vi "Where do VI's come from.vi"() -> ()   [LabVIEW 2015]
doc: "<<<<LabVIEW freeware>>>>\n\nFind the origin of all VIs in memory.\n\n<<<<LabVIEW freeware>>>>\n---------------------------------------\n(c) CIT Engineering NV\nKleinhoefstraat 6\nB-2440 Geel\nmailto: info@citeng.com\n---------------------------------------\nv1.1\nLV6i, 3D controls\nV1.0\nFirst release"
panel:
  in  "GetRunning":bool
  in  "Running VIs":i32(listbox)
  in  "Open":bool
  out "Current path":string
  in  "Delete":bool
  in  "Files not used in directory":i32[](listbox)
  in  "VIs":i32(listbox)
  in  "stop":bool
  in  "Paths":i32(listbox)
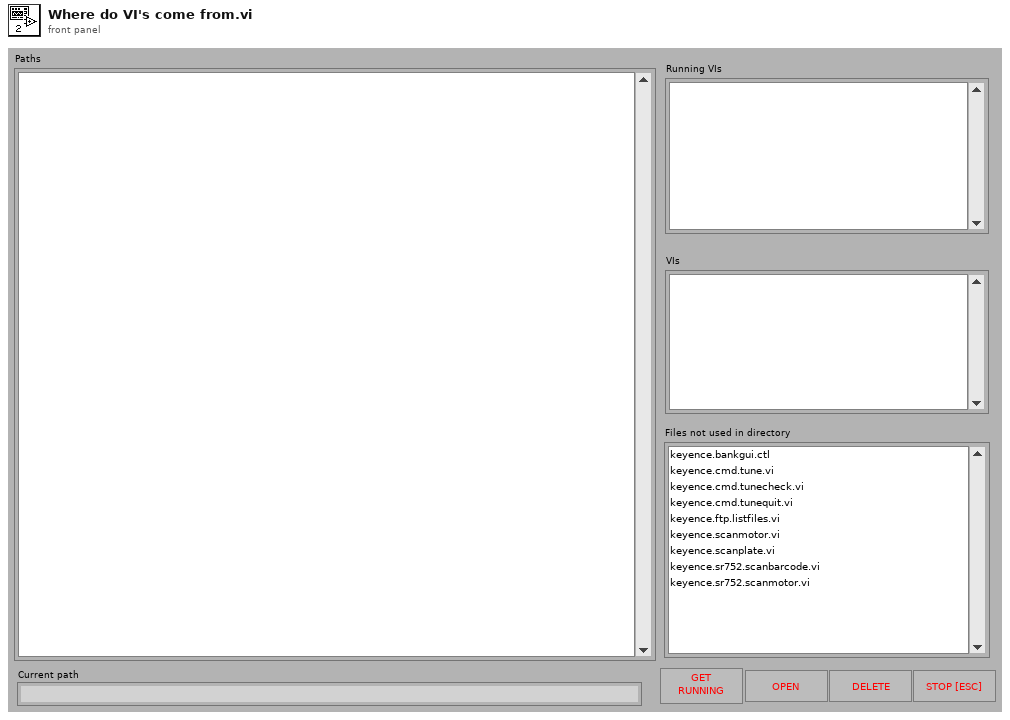
[diagram p1: front panel]
types:
  T1 = enum32{"Invalid", "Standard", "Closed", "Hidden", "Minimized", "Maximized"}
  T2 = cluster{"vi name":string, "vi path":path, "ds size":i32, "fpHeap size":i32, "bdHeap size":i32, "code size":i32, "callers":u32[], "callees":u32[]}[]
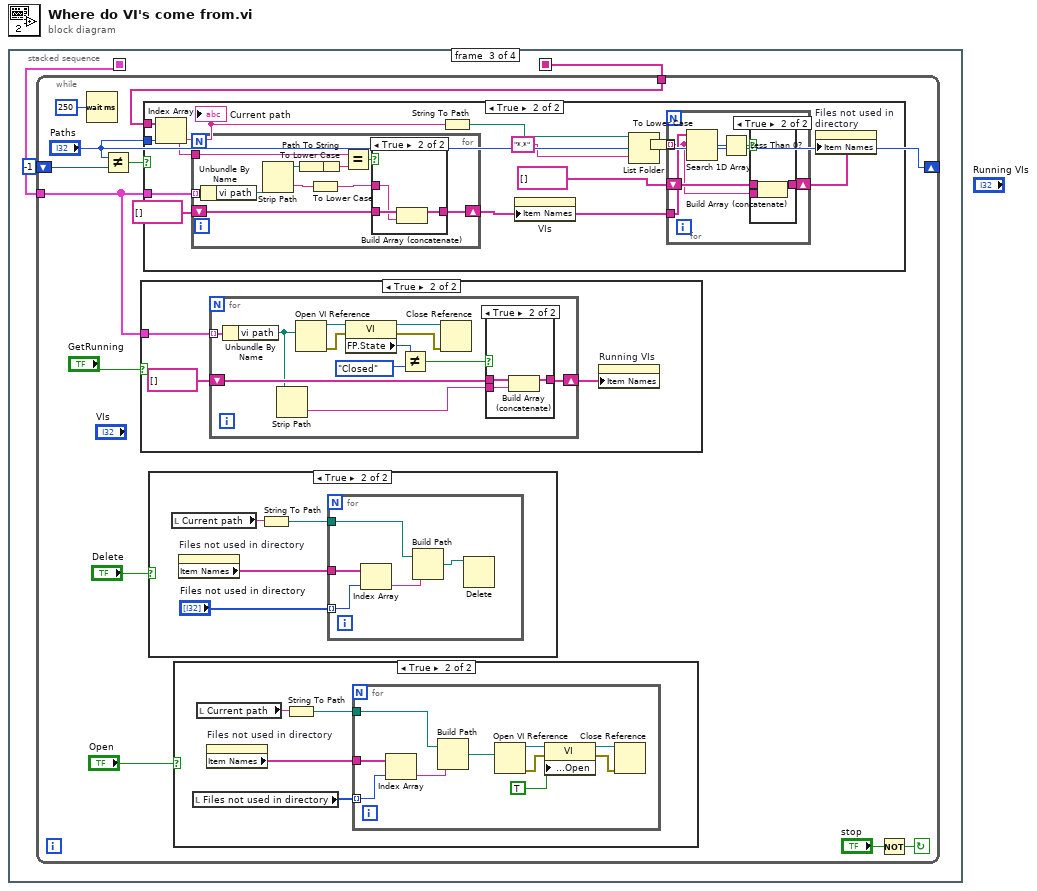
[diagram p0: block diagram]
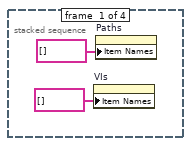
[diagram p2: hidden frame]
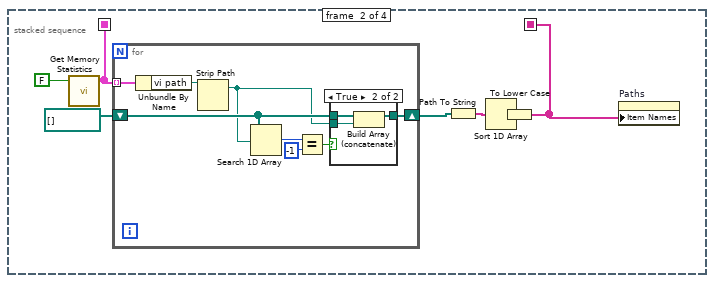
[diagram p3: hidden frame]
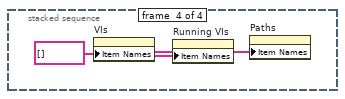
[diagram p12: hidden frame]
diagram:
  n1 = stacked-sequence {
    seq-local: [_ w3 _ _] -> [_ _ w24 _]
    seq-local: [_ w5 _ _] -> [_ _ w23 _]
    frame #0 {
      n2 = property on="VIs" class="LstBox (strict)"("Item Names"=string[] []) -> ()  [unwired: 2 in, 2 out]
      n3 = property on="Paths" class="LstBox (strict)"("Item Names"=string[] []) -> ()  [unwired: 2 in, 2 out]
    }
    frame #1 {
      n4 = call <vilib>:"Get Memory Statistics.vi"("get storage info? (T)"=FALSE) -> ("VI Memory Statistics"=w5:T2)  [unwired: 2 in, 2 out]
      n5 = for {
        tunnel: w5 -> [w17] mode=indexing
        shift-right: [w10] -> w8
        shift-left: path[] [] -> [w15]
        n6 = Unbundle By Name(w17) -> ("vi path"=w16:path)
        n7 = Strip Path(path=w16) -> (stripped path=w11:path)  [unwired: 1 out]
        n8 = Search 1D Array(1D array=w15, element=w11) -> (index of element=w14:i32)  [unwired: 1 in]
        n9 = Equal?(x=w14, y=-1) -> (x = y?=w12:bool)
        n10 = case shown="True" w12 {
          tunnel: w15 -> [w18 w21]
          tunnel: w11 -> [_ w20]
          tunnel: [w18 w19] -> w10
          frame False {
          }
          frame True {
            n11 = Build Array (concatenate)(w21, w20) -> (w19:path[])
          }
        }
      }
      n12 = Path To String(path=w8) -> (string=w7:string[])
      n13 = Sort 1D Array(array=w7) -> (sorted array=w6:string[])
      n14 = To Lower Case(string=w6) -> (all lower case string=w3:string[])
      n15 = property on="Paths" class="LstBox (strict)"("Item Names"=w3) -> ()  [unwired: 2 in, 2 out]
    }
    frame #2 {
      n16 = while {
        shift-left: -1 -> [w30]
        shift-right: ["Paths"] -> _
        tunnel: w23 -> [w26]
        tunnel: w24 -> [w33]
        stop <- w34 continue-if-true
        n17 = Wait (ms)(milliseconds to wait=u32 250) -> ()  [unwired: 1 out]
        n18 = Not Equal?(x="Paths", y=w30) -> (x != y?=w29:bool)
        n19 = case shown="True" "GetRunning" {
          tunnel: w26 -> [_ w36]
          frame False {
          }
          frame True {
            n20 = for {
              tunnel: w36 -> [w46] mode=indexing
              shift-right: [w39] -> w38
              shift-left: string[] [] -> [w45]
              n21 = Unbundle By Name(w46) -> ("vi path"=w41:path)
              n22 = Strip Path(path=w41) -> (name=w40:string)  [unwired: 1 out]
              n23 = Open VI Reference(vi path=w41) -> (vi reference=w50:refnum<vi>, error out=w49:errorcluster)  [unwired: 5 in]
              n24 = property class="VI"(reference=w50, error in=w49) -> (reference out=w47:refnum<vi>, error out=w48:errorcluster, "FP.State"=w44:T1)
              n25 = Not Equal?(x=w44, y=T1."Closed" ("Front Panel Window:State")) -> (x != y?=w42:bool)
              n26 = Close Reference(reference=w47, error in (no error)=w48) -> ()  [unwired: 1 out]
              n27 = case shown="True" w42 {
                tunnel: [w51 w53] -> w39
                tunnel: w45 -> [w51 w54]
                tunnel: w40 -> [_ w52]
                frame False {
                }
                frame True {
                  n28 = Build Array (concatenate)(w54, w52) -> (w53:string[])
                }
              }
            }
            n29 = property on="Running VIs" class="LstBox (strict)"("Item Names"=w38) -> ()  [unwired: 2 in, 2 out]
          }
        }
        n30 = case shown="True" w29 {
          tunnel: "Paths" -> [_ w89]
          tunnel: w33 -> [_ w88]
          tunnel: w26 -> [_ w79]
          frame False {
          }
          frame True {
            n31 = Index Array(array=w88, index=w89) -> (element=w86:string)
            "Current path" <- w86
            n32 = for {
              tunnel: w79 -> [w110] mode=indexing
              tunnel: w86 -> [w103]
              shift-right: [w106] -> w87
              shift-left: string[] [] -> [w105]
              n33 = Unbundle By Name(w110) -> ("vi path"=w109:path)
              n34 = Strip Path(path=w109) -> (stripped path=w108:path, name=w104:string)
              n35 = Path To String(path=w108) -> (string=w102:string)
              n36 = To Lower Case(string=w104) -> (all lower case string=w100:string)
              n37 = To Lower Case(string=w102) -> (all lower case string=w101:string)
              n38 = Equal?(x=w103, y=w101) -> (x = y?=w107:bool)
              n39 = case shown="True" w107 {
                tunnel: [w111 w112] -> w106
                tunnel: w105 -> [w111 w114]
                tunnel: w100 -> [_ w113]
                frame False {
                }
                frame True {
                  n40 = Build Array (concatenate)(w114, w113) -> (w112:string[])
                }
              }
            }
            n41 = String To Path(string=w86) -> (path=w85:path)
            n42 = property on="VIs" class="LstBox (strict)"("Item Names"=w87) -> ()  [unwired: 2 in, 2 out]
            n43 = List Folder(path=w85, pattern="*.*") -> (filenames=w83:string[])  [unwired: 2 in, 3 out]
            n44 = To Lower Case(string=w83) -> (all lower case string=w80:string[])
            n45 = for {
              tunnel: w80 -> [w91] mode=indexing
              tunnel: w87 -> [w95]
              shift-right: [w90] -> w81
              shift-left: string[] [] ("Item Names") -> [w92]
              n46 = Search 1D Array(1D array=w95, element=w91) -> (index of element=w94:i32)  [unwired: 1 in]
              n47 = Less Than 0?(x=w94) -> (x < 0?=w93:bool)
              n48 = case shown="True" w93 {
                tunnel: w92 -> [w96 w99]
                tunnel: w91 -> [_ w98]
                tunnel: [w96 w97] -> w90
                frame False {
                }
                frame True {
                  n49 = Build Array (concatenate)(w99, w98) -> (w97:string[])
                }
              }
            }
            n50 = property on="Files not used in directory" class="LstBox (strict)"("Item Names"=w81) -> ()  [unwired: 2 in, 2 out]
          }
        }
        n51 = case shown="True" "Delete" {
          frame False {
          }
          frame True {
            n52 = local read "Current path"() -> (w72:string)
            n53 = property on="Files not used in directory" class="LstBox (strict)"() -> ("Item Names"=w71:string[])  [unwired: 2 in, 2 out]
            n54 = String To Path(string=w72) -> (path=w69:path)
            n55 = for {
              tunnel: w71 -> [w77]
              tunnel: "Files not used in directory" -> [w76] mode=indexing
              tunnel: w69 -> [w75]
              n56 = Index Array(array=w77, index=w76) -> (element=w74:string)
              n57 = Build Path(base path=w75, name or relative path=w74) -> (appended path=w73:path)
              n58 = Delete(path (use dialog)=w73) -> ()  [unwired: 4 in, 3 out]
            }
          }
        }
        n59 = case shown="True" "Open" {
          frame False {
          }
          frame True {
            n60 = local read "Files not used in directory"() -> (w55:i32[])
            n61 = local read "Current path"() -> (w58:string)
            n62 = property on="Files not used in directory" class="LstBox (strict)"() -> ("Item Names"=w56:string[])  [unwired: 2 in, 2 out]
            n63 = String To Path(string=w58) -> (path=w57:path)
            n64 = for {
              tunnel: w56 -> [w68]
              tunnel: w55 -> [w67] mode=indexing
              tunnel: w57 -> [w66]
              n65 = Index Array(array=w68, index=w67) -> (element=w65:string)
              n66 = Build Path(base path=w66, name or relative path=w65) -> (appended path=w64:path)
              n67 = Open VI Reference(vi path=w64) -> (vi reference=w63:refnum<vi>, error out=w61:errorcluster)  [unwired: 5 in]
              n68 = property class="VI"(reference=w63, error in=w61, "Front Panel Window:Open"=TRUE) -> (reference out=w59:refnum<vi>, error out=w60:errorcluster)
              n69 = Close Reference(reference=w59, error in (no error)=w60) -> ()  [unwired: 1 out]
            }
          }
        }
        n70 = Not(x="stop") -> (.not. x?=w34:bool)
      }
    }
    frame #3 {
      w115 = string[] [] ("Item Names")
      n71 = property on="VIs" class="LstBox (strict)"("Item Names"=w115) -> ()  [unwired: 2 in, 2 out]
      n72 = property on="Running VIs" class="LstBox (strict)"("Item Names"=w115) -> ()  [unwired: 2 in, 2 out]
      n73 = property on="Paths" class="LstBox (strict)"("Item Names"=w115) -> ()  [unwired: 2 in, 2 out]
    }
  }
